vi "Read Start A-Scan Array.vi"(8 "error in (no error)":errorcluster, 11 "NuFern in":refnum<class "NuFern.lvclass">) -> (0 "error out":errorcluster, 2 "Start A-Scan Array":u32[](array[numeric]), 3 "NuFern out":refnum<class "NuFern.lvclass">)   [LabVIEW 2015, in "NuFern.lvclass"]
uses:
  NuFern.lvclass
  NuFern.lvclass/NuFern.ctl
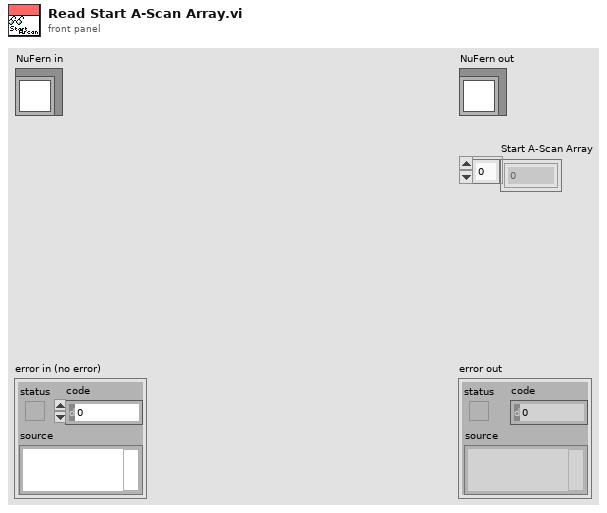
[diagram p1: front panel]
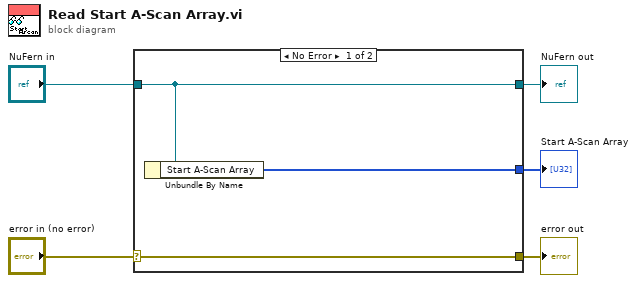
[diagram p0: block diagram]
diagram:
  n1 = case shown="No Error" "error in (no error)" {
    selector: "error in (no error)" -> [w8 w9]
    tunnel: [w8 w9] -> w4
    tunnel: [w7 w10] -> w2
    tunnel: "NuFern in" -> [w7 w10]
    tunnel: [w6 _] -> w1
    frame No Error {
      n2 = Unbundle By Name(w7) -> ("Start A-Scan Array"=w6:u32[])
    }
    frame Error {
    }
  }
  "error out" <- w4
  "NuFern out" <- w2
  "Start A-Scan Array" <- w1
